vi "Cancel Calling VI Wnd Topmost.vi"(8 "Error In":errorcluster) -> (0 "Error Out":errorcluster)   [LabVIEW 2020]
doc: "Sets the Caller VIs front panel NoTopmost (above all non-topmost windows), thereby cancelling the TopMost setting.\n\nCopyright © 2010 Blue Ridge Test, Inc.\nwww.BlueRidgeTest.com"
uses:
  USER32.DLL
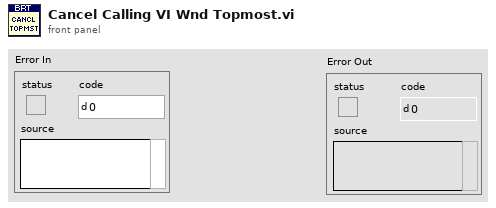
[diagram p1: front panel]
types:
  T1 = enum32{"Invalid", "Standard", "Closed", "Hidden", "Minimized", "Maximized"}
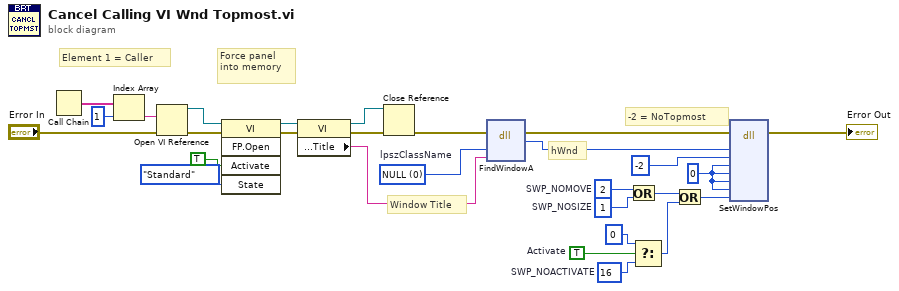
[diagram p0: block diagram]
diagram:
  w5 = TRUE  # Activate
  w6 = u32 2  # SWP_NOMOVE
  w7 = u32 1  # SWP_NOSIZE
  w8 = u32 16  # SWP_NOACTIVATE
  w4 = 0
  w26 = 0 items=["NULL"]  # lpszClassName
  # "-2 = NoTopmost"
  # "hWnd"
  # "Force panel\ninto memory"
  # "Window Title"
  # "Element 1 = Caller"
  n1 = Call Chain() -> (call chain=w24:string[])
  n2 = Index Array(array=w24, index=1) -> (element=w23:string)
  n3 = Open VI Reference(vi path=w23, error in (no error)="Error In") -> (vi reference=w20:refnum<vi>, error out=w21:errorcluster)  [unwired: 4 in]
  n4 = invoke class="VI" method="FP.Open"(reference=w20, error in=w21, "Activate"=TRUE ("Activate?"), "State"=T1."Standard") -> (reference out=w18:refnum<vi>, error out=w19:errorcluster)  [unwired: 1 in, 3 out]
  n5 = property class="VI"(reference=w18, error in=w19) -> (reference out=w16:refnum<vi>, error out=w15:errorcluster, "Front Panel.Title"=w17:string)
  n6 = Close Reference(reference=w16, error in (no error)=w15) -> (error out=w14:errorcluster)
  n7 = dll-call lib="USER32.DLL" fn="FindWindowA" label="FindWindow"(error in=w14, "lpszClassName"=w26, "lpszWindowName"=w17) -> (error out=w3:errorcluster, "hWnd"=w2:u32)  [unwired: 4 in, 1 out]
  n8 = Or(x=w6, y=w7) -> (x .or. y?=w11:u32)
  n9 = Select(t=u32 0, s=w5, f=w8) -> (s? t:f=w10:u32)
  n10 = Or(x=w11, y=w10) -> (x .or. y?=w12:u32)
  n11 = dll-call lib="USER32.DLL" fn="SetWindowPos"(error in=w3, "hWnd"=w2, "hWndInsertAfter"=-2, "left"=w4, "top"=w4, "width"=w4, "height"=w4, "fuFlags"=w12) -> (error out=→"Error Out":errorcluster)  [unwired: 8 in, 3 out]
